vi "Read U8 Array External.vi"(7 "Channel Index":i32, 8 "error in (no error)":errorcluster, 9 "Timeout (ms)":i32, 11 "CIFCorePlugin in":refnum<class "CIFCorePlugin.lvclass">) -> (0 "error out":errorcluster, 1 "timed out?":bool, 2 "U8 With Header":u8[](array[numeric]) format="%.0x", 3 "CIFCorePlugin out":refnum<class "CIFCorePlugin.lvclass">, 4 "Header":T1)   [LabVIEW 2021, in "CIFCorePlugin.lvclass"]
doc: "Read the full payload bytes, including the encoded header. This is intended for advanced applications where the full buffer will be sent externally."
uses:
  CIFCorePlugin.lvclass
  CIFCorePlugin.lvclass/CIFCorePlugin.ctl
  <vilib>/CIF Foundation/CIF Channels Core/CIFChannels/CIFChannels.lvclass
  <vilib>/CIF Foundation/CIF Channels Core/ChannelCommon/typedef/FIFO Header.ctl
  <vilib>/CIF Foundation/CIF Channels Core/ChannelCommon/ChannelCommon.lvlib
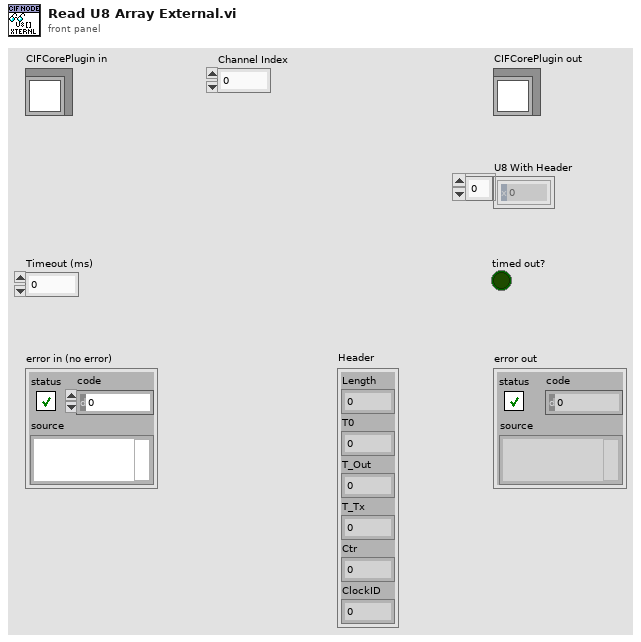
[diagram p1: front panel]
types:
  T1 = typedef "ChannelCommon.lvlib/FIFO Header.ctl" = cluster{"Length":u64, "T0":i64, "T_Out":i64, "T_Tx":i64, "Ctr":u64, "ClockID":u8}
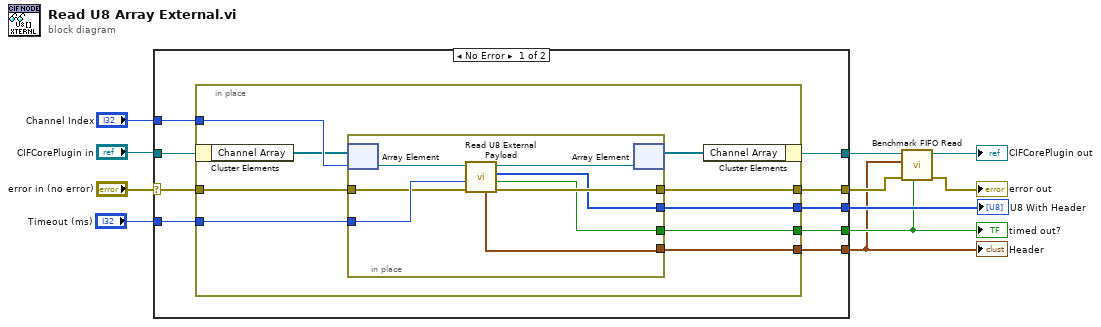
[diagram p0: block diagram]
diagram:
  n1 = case shown="No Error" "error in (no error)" {
    selector: "error in (no error)" -> [w20 w39]
    tunnel: [w19 w39] -> w4
    tunnel: [w16 w38] -> w6
    tunnel: "CIFCorePlugin in" -> [w17 w38]
    tunnel: [w18 _] -> w7
    tunnel: "Channel Index" -> [w15 _]
    tunnel: "Timeout (ms)" -> [w14 _]
    tunnel: [w13 _] -> w2
    tunnel: [w12 _] -> w1
    frame No Error {
      n2 = in-place {
        in-place-border: w20 -> [w21]
        in-place-border: [w22] -> w19
        in-place-border: [w29] -> w18
        in-place-border: w15 -> [w28]
        in-place-border: w14 -> [w27]
        in-place-border: [w26] -> w13
        in-place-border: [w25] -> w12
        n3 = in-place-cluster #1(w17) -> ("Channel Array"=w24:refnum<class "CIFChannels.lvclass">[])
        n4 = in-place {
          in-place-border: w21 -> [w35]
          in-place-border: [w33] -> w22
          in-place-border: [w31] -> w29
          in-place-border: w27 -> [w36]
          in-place-border: [w32] -> w26
          in-place-border: [w34] -> w25
          n5 = in-place-array #2(w24, w28) -> (w37:refnum<class "CIFChannels.lvclass">)
          n6 = call-dynamic "Read U8 External Payload.vi"("error in (no error)"=w35, "Timeout (ms)"=w36, "CIFChannels in"=w37) -> ("error out"=w33:errorcluster, "timed out?"=w32:bool, "Data out"=w31:u8[], "CIFChannels out"=w30:refnum<class "CIFChannels.lvclass">, "Header"=w34:T1)  [unwired: 4 in]
          n7 = in-place-array #2(w30) -> (w23:refnum<class "CIFChannels.lvclass">[])  [unwired: 1 out]
        }
        n8 = in-place-cluster #1("Channel Array"=w23) -> (w16:refnum<class "CIFCorePlugin.lvclass">)
      }
    }
    frame Error {
    }
  }
  "timed out?" <- w2
  "Header" <- w1
  "U8 With Header" <- w7
  n9 = call "Benchmark FIFO Read.vi"("timed out?"=w2, "error in (no error)"=w4, "Header"=w1, "CIFCorePlugin in"=w6) -> ("error out"=→"error out":errorcluster, "CIFCorePlugin out"=→"CIFCorePlugin out":refnum<class "CIFCorePlugin.lvclass">)  [unwired: 6 in]
